vi "configure.vi"(8 "error in (no error)":errorcluster, 11 "GenericPlugin in":refnum<class "ScanHeadMH100729FPGA.lvclass">) -> (0 "error out":errorcluster, 3 "GenericPlugin out":refnum<class "ScanHeadMH100729FPGA.lvclass">)   [LabVIEW 2010, in "ScanHeadMH100729FPGA.lvclass"]
doc: "The dynamic dispatch version of this VI loads and displays the configuration file associated with the plug-in object. The user modify and save the configuration data."
uses:
  ScanHeadMH100729FPGA.lvclass
  common/xcontrols/XComponentSpecification/XComponentSpecification/XComponentSpecification.xctl
  ScanHeadMH100729FPGA.lvclass/ScanHeadMH100729FPGA.ctl
  AnalogOut/GenericAnalogOut/GenericAnalogOut/GenericAnalogOut.lvclass
  common/classes/ErrorController/ErrorController/class_data.vi
  common/classes/GenericComponent/GenericComponent/GenericComponent.lvclass
  common/classes/ErrorController/ErrorController/ErrorController.lvclass
panel:
  in  "cancel":bool
  in  "save":bool
  out "Configuration":string
  in  "Tab Control":enum32{"intensity modifier"}(tab)
  in  "modifier factor":dbl[unit] caption="translation factor"
  in  "intensity modifier spec":T1(xcontrol)
  # "Configure ScanHeadMH100729FPGA"
  # "Here, you can modify a component of type AnalogOut, which controls a laser-beam intensity modifier such as a Pockels cell.\n\nLeave empty if not needed. \n\nThe translation factor specifies how an intensity value is translated into a voltage that is provided to the intensity modifier.\nExample: 100% should correspond to 1.00V provided to a Pockels cell modulator; this would require the translation factor to be 0.01."
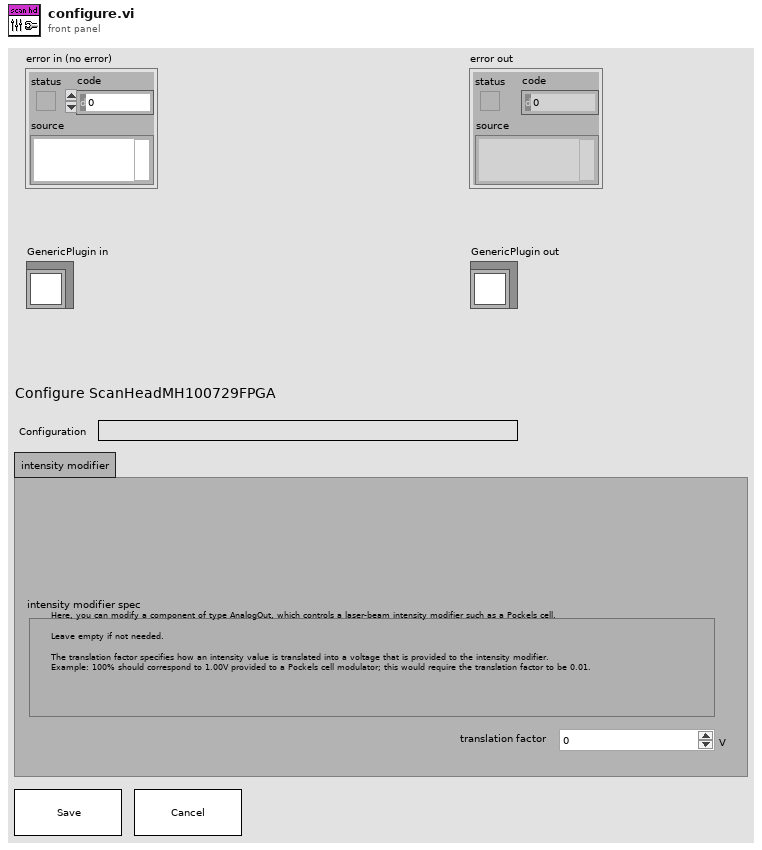
[diagram p1: front panel]
types:
  T1 = cluster{"class path":string, "configuration":string, "label":string, "settings name":string}
  T2 = typedef "plugin_specification.ctl" = cluster{"class path":string, "configuration":string, "label":string, "settings name":string}
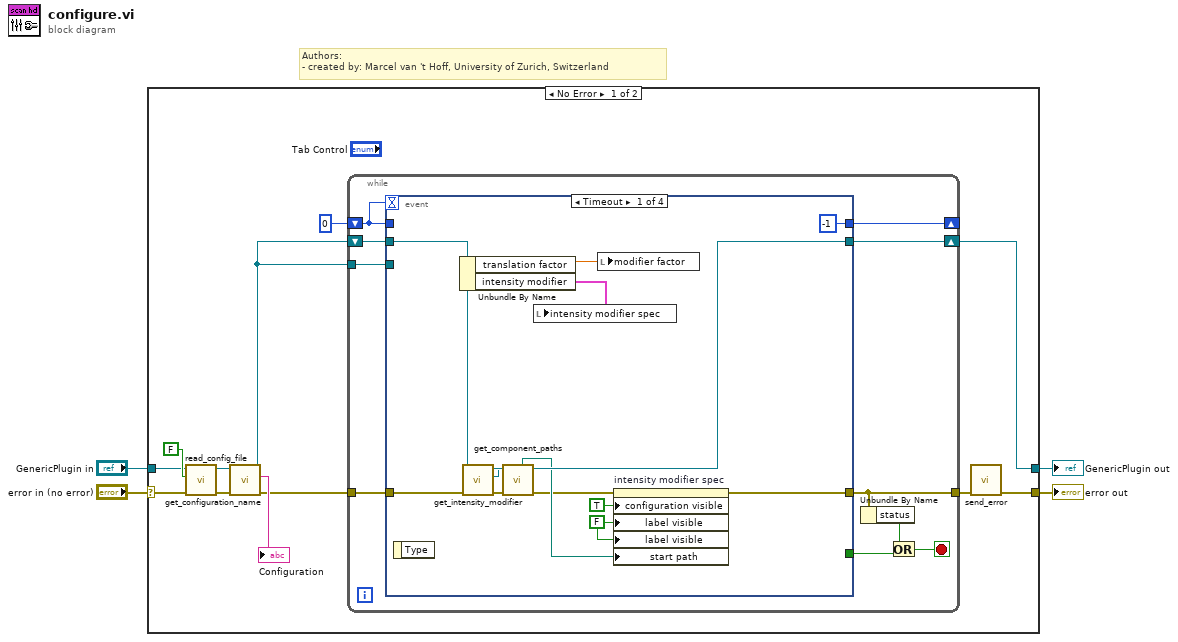
[diagram p0: block diagram]
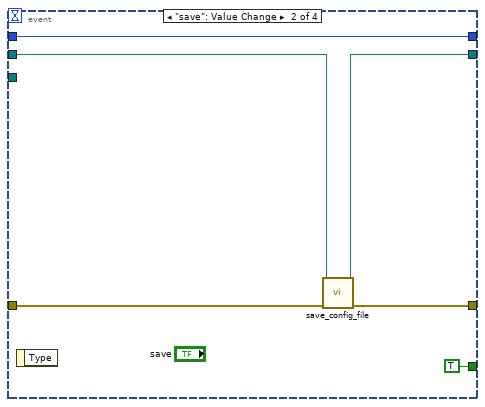
[diagram p2: hidden frame]
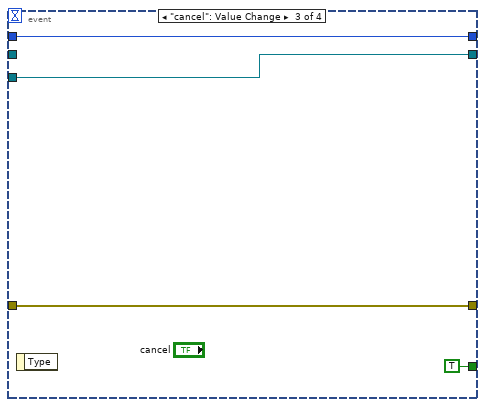
[diagram p3: hidden frame]
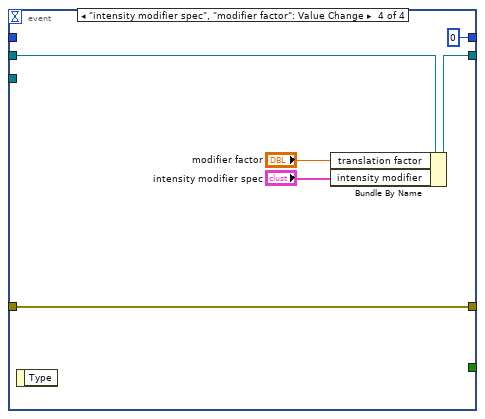
[diagram p4: hidden frame]
diagram:
  # "Authors: \n- created by: Marcel van 't Hoff, University of Zurich, Switzerland"
  n1 = case shown="No Error" "error in (no error)" {
    selector: "error in (no error)" -> [w11 w57]
    tunnel: "GenericPlugin in" -> [w13 w56]
    tunnel: [w7 w57] -> w2
    tunnel: [w10 w56] -> w1
    frame No Error {
      n2 = call-dynamic "read_config_file.vi"("error in (no error)"=w11, "force load?"=FALSE, "GenericPlugin in"=w13) -> ("error out"=w15:errorcluster, "GenericPlugin out"=w16:refnum<class "ScanHeadMH100729FPGA.lvclass">)  [unwired: 7 out]
      n3 = call "get_configuration_name.vi"("error in (no error)"=w15, "GenericPlugin.lvclass in"=w16) -> ("error out"=w9:errorcluster, "configuration name"=→"Configuration":string, "GenericPlugin.lvclass out"=w5:refnum<class "ScanHeadMH100729FPGA.lvclass">)  [unwired: 7 in]
      n4 = while {
        tunnel: w9 -> [w24]
        tunnel: [w23] -> w6
        shift-right: [w19] -> _
        shift-left: 0 -> [w18]
        shift-right: [w25] -> w10
        shift-left: w5 -> [w26]
        tunnel: w5 -> [w17]
        stop <- w21 stop-if-true
        n5 = event shown="[0] Timeout" {
          selector: _ -> [_ _ _ _]
          dyn-events: _ -> [_ _ _ _]
          timeout: w18 -> [_ _ _ _]
          tunnel: [w37 w41 w47 w52] -> w25
          tunnel: w26 -> [w32 w42 _ w53]
          tunnel: [w28 w43 w49 w55] -> w23
          tunnel: w24 -> [w34 w44 w49 w55]
          tunnel: [_ TRUE TRUE _] -> w20
          tunnel: [-1 w40 w46 0] -> w19
          tunnel: w18 -> [_ w40 w46 _]
          tunnel: w17 -> [_ _ w47 _]
          event Timeout {
            w30 = FALSE ("label visible")
            n6 = event-data() -> ()  [unwired: 1 in, 1 out]
            n7 = Unbundle By Name(w32) -> ("translation factor"=w38:dbl[unit], "intensity modifier"=w33:T2)
            n8 = call-dynamic "get_intensity_modifier.vi"("error in (no error)"=w34, "ScanHeadMH100729FPGA in"=w32) -> ("error out"=w36:errorcluster, "intensity modifier"=w35:refnum<class "GenericAnalogOut.lvclass">, "ScanHeadMH100729FPGA out"=w37:refnum<class "ScanHeadMH100729FPGA.lvclass">)  [unwired: 7 in]
            n9 = call-dynamic "get_component_paths.vi"("error in (no error)"=w36, "GenericComponent in"=w35) -> ("error out"=w27:errorcluster, "component type directory"=w29:path)  [unwired: 4 in, 4 out]
            n10 = local write "intensity modifier spec"(w33) -> ()
            n11 = local write "modifier factor"(w38) -> ()
            n12 = property on="intensity modifier spec" class="XComponentSpecification (strict"(error in=w27, "configuration visible"=TRUE, "label visible"=w30, "label visible"=w30, "start path"=w29) -> (error out=w28:errorcluster)  [unwired: 1 in, 1 out]
          }
          event "save": Value Change {
            n13 = event-data() -> ()  [unwired: 1 in, 1 out]
            n14 = call-dynamic "save_config_file.vi"("error in (no error)"=w44, "GenericPlugin in"=w42) -> ("error out"=w43:errorcluster, "GenericPlugin out"=w41:refnum<class "ScanHeadMH100729FPGA.lvclass">)  [unwired: 2 in, 6 out]
          }
          event "cancel": Value Change {
            n15 = event-data() -> ()  [unwired: 1 in, 1 out]
          }
          event "intensity modifier spec", "modifier factor": Value Change {
            n16 = event-data() -> ()  [unwired: 1 in, 1 out]
            n17 = Bundle By Name(cluster=w53, "translation factor"="modifier factor", "intensity modifier"="intensity modifier spec") -> (w52:refnum<class "ScanHeadMH100729FPGA.lvclass">)
          }
        }
        n18 = Unbundle By Name(w23) -> ("status"=w22:bool)
        n19 = Or(x=w22, y=w20) -> (x .or. y?=w21:bool)
      }
      n20 = call "send_error.vi"("error in (no error)"=w6) -> ("error out"=w7:errorcluster)  [unwired: 10 in]
    }
    frame Error {
    }
  }
  "error out" <- w2
  "GenericPlugin out" <- w1
